vi "lightsource-set.vi"(3 "Select NKT System":enum32{"SuperK Varia (VIS)", "Extend-UV"}(radio), 4 "Excitation Input":T2) -> (0 "PLE Measurment Finished?":bool, 1 "Excitation Input":T2, 2 "Wavelength Cluster":T1, 5 "Powermeter Wavelength (nm)":i32)   [LabVIEW 2017]
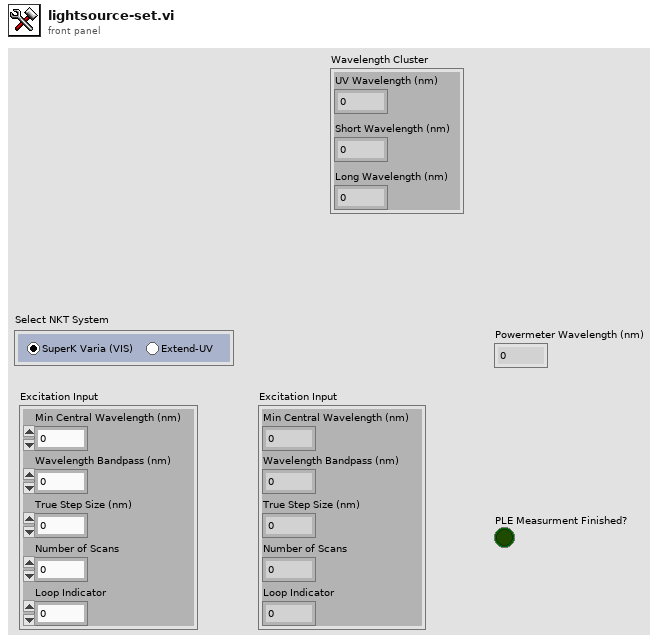
[diagram p1: front panel]
types:
  T1 = cluster{"UV Wavelength (nm)":i32, "Short Wavelength (nm)":dbl, "Long Wavelength (nm)":dbl}
  T2 = cluster{"Min Central Wavelength (nm)":i32, "Wavelength Bandpass (nm)":i32, "True Step Size (nm) ":i32, "Number of Scans":i32, "Loop Indicator":i32}
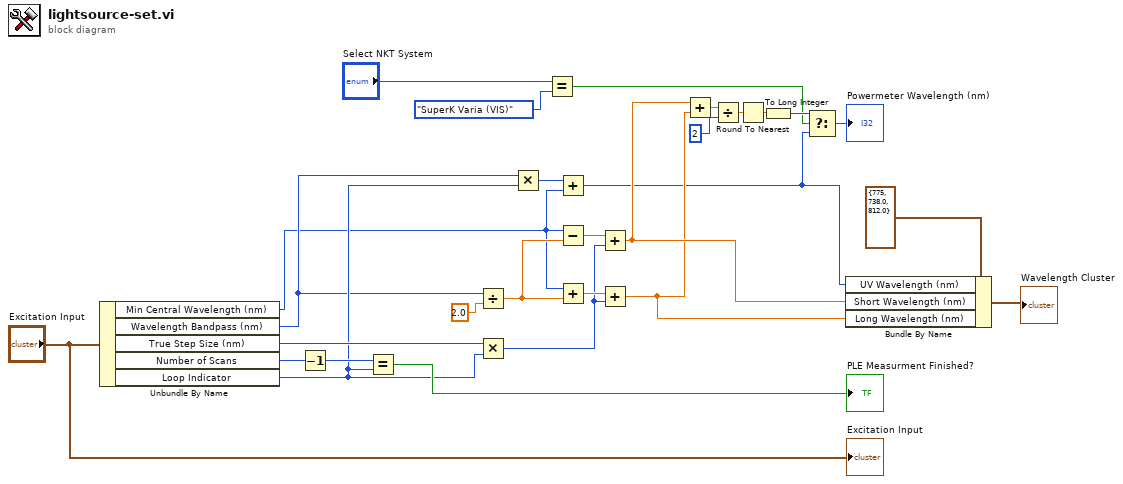
[diagram p0: block diagram]
diagram:
  n1 = Unbundle By Name("Excitation Input") -> ("Min Central Wavelength (nm)"=w13:i32, "Wavelength Bandpass (nm)"=w15:i32, "True Step Size (nm)"=w20:i32, "Number of Scans"=w24:i32, "Loop Indicator"=w16:i32)
  n2 = Decrement(x=w24) -> (x-1=w23:i32)
  n3 = Equal?(x=w23, y=w16) -> (x = y?=→"PLE Measurment Finished?":bool)
  n4 = Divide(x=w15, y=2.0) -> (x/y=w27:dbl)
  n5 = Multiply(x=w20, y=w16) -> (x*y=w21:i32)
  n6 = Multiply(x=w15, y=w16) -> (x*y=w14:i32)
  n7 = Equal?(x="Select NKT System", y=enum32{"SuperK Varia (VIS)", "Extend-UV"}."SuperK Varia (VIS)" ("Select NKT System")) -> (x = y?=w8:bool)
  n8 = Add(x=w14, y=w13) -> (x+y=w1:i32)
  n9 = Subtract(x=w13, y=w27) -> (x-y=w26:dbl)
  n10 = Add(x=w13, y=w27) -> (x+y=w25:dbl)
  n11 = Add(x=w26, y=w21) -> (x+y=w4:dbl)
  n12 = Add(x=w25, y=w21) -> (x+y=w3:dbl)
  n13 = Add(x=w4, y=w3) -> (x+y=w18:dbl)
  n14 = Divide(x=w18, y=2) -> (x/y=w7:dbl)
  n15 = Round To Nearest(number=w7) -> (nearest integer value=w6:dbl)
  n16 = To Long Integer(number=w6) -> (32bit integer=w12:i32)
  n17 = Select(t=w12, s=w8, f=w1) -> (s? t:f=→"Powermeter Wavelength (nm)":i32)
  n18 = Bundle By Name(cluster=T1 {"UV Wavelength (nm)"=775, "Short Wavelength (nm)"=738.0, "Long Wavelength (nm)"=812.0} ("Wavelength Cluster"), "UV Wavelength (nm)"=w1, "Short Wavelength (nm)"=w4, "Long Wavelength (nm)"=w3) -> (→"Wavelength Cluster":T1)
  "Excitation Input" <- "Excitation Input"
